vi "Get Request.vi"(11 "SSE Client in":refnum<class "SSE Client.lvclass">) -> (2 "Request":refnum<class "Request.lvclass">, 3 "SSE Client out":refnum<class "SSE Client.lvclass">)   [LabVIEW 2020, in "HTTP Server.lvlib" / "SSE Client.lvclass"]
uses:
  SSE Client.lvclass
  SSE Client.lvclass/SSE Client.ctl
  lv-http-util/HTTP Utils/Request/Request.lvclass
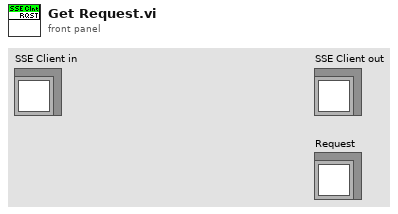
[diagram p1: front panel]
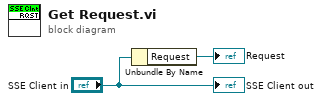
[diagram p0: block diagram]
diagram:
  n1 = Unbundle By Name("SSE Client in") -> ("Request"=→"Request":refnum<class "Request.lvclass">)
  "SSE Client out" <- "SSE Client in"
